vi "ReadHdrDates_LS1.vi"(7 "Data Folder Path":path, 8 "error in (no error)":errorcluster, 9 "Session":i32=-1, 10 "Date String":string="All" caption="Date String (yymmdd)", 11 "nombre (-1)":i32=-1) -> (0 "error out":errorcluster, 2 "Dates":string[](array[string]), 3 "ScanParams":T1[](array[typedef]))   [LabVIEW 2010]
doc: "Ce VI lit les données contenu dans le fichier de sauvegarde automatique. Ces données correspondent aux valeurs prises lors du dernier balayage. La sauvegarde automatique est effectué après chaque acquisition."
uses:
  Interface Class/ScanParams.ctl
  Interface Class/Interface.lvclass
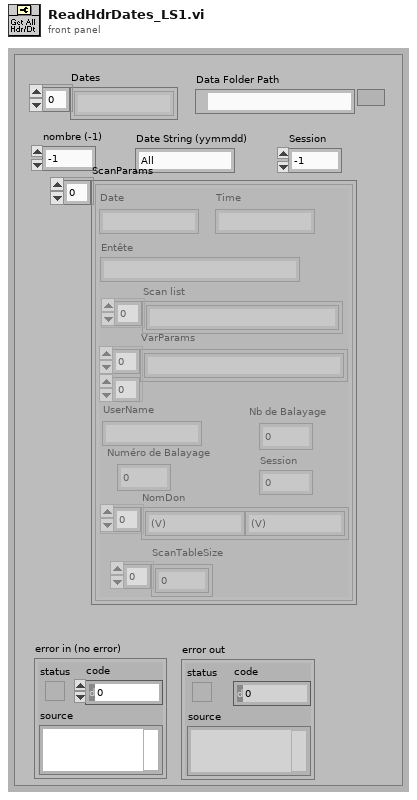
[diagram p1: front panel]
types:
  T1 = typedef "Interface.lvclass/ScanParams.ctl" = cluster{"Entête":string, "Scan list":string[], "NbCourbe":i32, "IndCourbe":i64, "NomDon":string[], "Session ":i32, "Date":string, "Time":string, "VarParams":string[][], "UserName":string, "ScanTableSize":i32[]}
  T2 = enum16{"open", "replace", "create", "open or create", "replace or create", "replace or create with confirmation"}
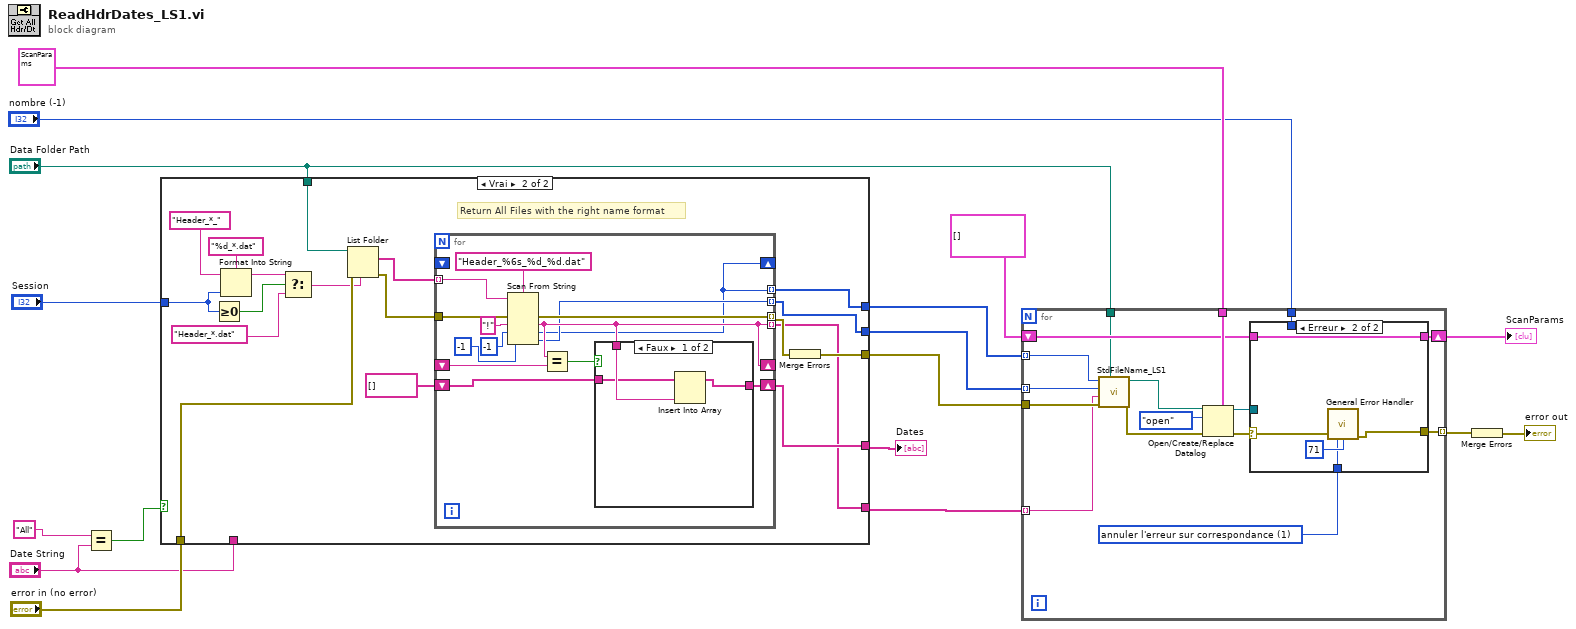
[diagram p0: block diagram]
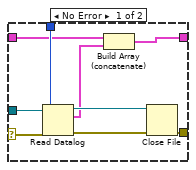
[diagram p2: hidden frame]
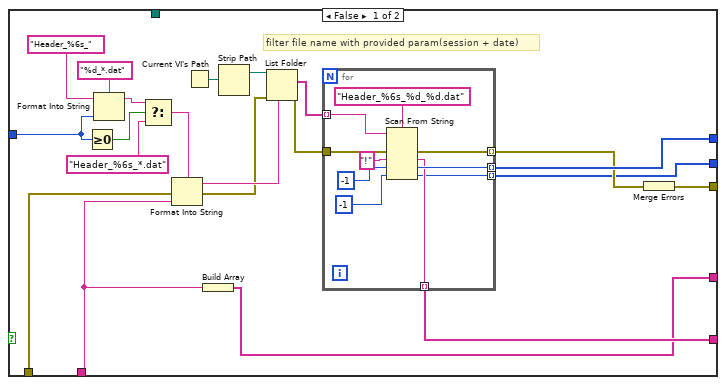
[diagram p3: hidden frame]
diagram:
  n1 = Equal?(x="All" ("Date String"), y="Date String") -> (x = y?=w8:bool)
  n2 = case shown="Vrai" w8 {
    tunnel: "error in (no error)" -> [w36 w66]
    tunnel: [w31 w61] -> w11
    tunnel: [w30 w64] -> w14
    tunnel: "Date String" -> [w27 _]
    tunnel: [w28 w59] -> w6
    tunnel: [w26 w60] -> w5
    tunnel: "Session" -> [w21 w54]
    tunnel: [w18 w50] -> w3
    tunnel: "Data Folder Path" -> [_ w49]
    frame False {
      # "filter file name with provided param(session + date)"
      n3 = Greater Or Equal To 0?(x=w21) -> (x >= 0?=w22:bool)
      n4 = Format Into String(format string="%d_*.dat" ("filtre"), initial string="Header_%6s_" ("filtre"), w21) -> (resulting string=w24:string)  [unwired: 1 in, 1 out]
      n5 = Select(t=w24, s=w22, f="Header_%6s_*.dat" ("filtre")) -> (s? t:f=w20:string)
      n6 = Format Into String(format string=w20, error in=w36, w27) -> (resulting string=w35:string, error out=w34:errorcluster)  [unwired: 1 in]
      n7 = Current VI's Path() -> (path=w38:path)
      n8 = Build Array(w27) -> (w26:string[])
      n9 = Strip Path(path=w38) -> (stripped path=w37:path)  [unwired: 1 out]
      n10 = List Folder(path=w37, pattern=w35, error in=w34) -> (filenames=w33:string[], error out=w32:errorcluster)  [unwired: 1 in, 2 out]
      n11 = for {
        tunnel: w33 -> [w48] mode=indexing
        tunnel: w32 -> [w47]
        tunnel: [w46] -> w29 mode=indexing
        tunnel: [w43] -> w31 mode=indexing
        tunnel: [w42] -> w28 mode=indexing
        tunnel: [w40] -> w18 mode=indexing
        n12 = Scan From String(format string="Header_%6s_%d_%d.dat" ("chaîne de format"), input string=w48, error in=w47, default 1="!" ("valeur par défaut 1"), default 2=-1 ("Session"), default 3=i64 -1 ("valeur par défaut 3")) -> (error out=w46:errorcluster, output 1=w42:string, output 2=w43:i32, output 3=w40:i64)  [unwired: 1 in, 2 out]
      }
      n13 = Merge Errors(w29) -> (w30:errorcluster)
    }
    frame True {
      # "Return All Files with the right name format"
      n14 = Greater Or Equal To 0?(x=w54) -> (x >= 0?=w55:bool)
      n15 = Format Into String(format string="%d_*.dat" ("filtre"), initial string="Header_*_" ("filtre"), w54) -> (resulting string=w56:string)  [unwired: 1 in, 1 out]
      n16 = Select(t=w56, s=w55, f="Header_*.dat" ("filtre")) -> (s? t:f=w52:string)
      n17 = List Folder(path=w49, pattern=w52, error in=w66) -> (filenames=w65:string[], error out=w51:errorcluster)  [unwired: 1 in, 2 out]
      n18 = for {
        tunnel: w65 -> [w80] mode=indexing
        tunnel: w51 -> [w79]
        tunnel: [w78] -> w63 mode=indexing
        shift-right: [w70] -> _
        shift-left: _ -> [w73]
        shift-right: [w71] -> w60
        shift-left: string[] [] ("tableau") -> [w72]
        tunnel: [w68] -> w61 mode=indexing
        tunnel: [w70] -> w59 mode=indexing
        tunnel: [w69] -> w50 mode=indexing
        shift-right: [w68] -> _
        shift-left: _ -> [_]
        n19 = Scan From String(format string="Header_%6s_%d_%d.dat" ("chaîne de format"), input string=w80, error in=w79, default 1="!" ("valeur par défaut 1"), default 2=-1 ("Session"), default 3=i64 -1 ("Session")) -> (error out=w78:errorcluster, output 1=w70:string, output 2=w68:i32, output 3=w69:i64)  [unwired: 1 in, 2 out]
        n20 = Equal?(x=w70, y=w73) -> (x = y?=w74:bool)
        n21 = case shown="Faux" w74 {
          tunnel: w70 -> [w83 _]
          tunnel: w72 -> [w82 w84]
          tunnel: [w81 w84] -> w71
          frame False {
            n22 = Insert Into Array(array=w82, new element=w83) -> (w81:string[])  [unwired: 1 in]
          }
          frame True {
          }
        }
      }
      n23 = Merge Errors(w63) -> (w64:errorcluster)
    }
  }
  "Dates" <- w5
  n24 = for {
    tunnel: [w100] -> w13 mode=indexing
    tunnel: T1 {"Entête"="", "Scan list"=[], "NbCourbe"=1, "IndCourbe"=1, "NomDon"=["RTêta;", "X&Y;"], "Session "=0, "Date"="", "Time"="", "VarParams"=[], "UserName"="", "ScanTableSize"=[]} ("ScanParams") -> [w99]
    tunnel: w6 -> [w89] mode=indexing
    tunnel: "nombre (-1)" -> [w94]
    tunnel: w14 -> [w93]
    tunnel: w11 -> [w92] mode=indexing
    shift-right: [w90] -> w2
    shift-left: T1[] [] -> [w91]
    tunnel: w3 -> [w88] mode=indexing
    tunnel: "Data Folder Path" -> [w87]
    w85 = 1 items=["pas d'exception", "annuler l'erreur sur correspondance", "définir l'erreur sur correspondance"] ("[exception action] (none:0)")
    n25 = call "StdFileName_LS1.vi"("chemin de base"=w87, "error in (no error)"=w93, "Date"=w89, "Scan"=w88, "Session"=w92) -> ("error out"=w97:errorcluster, "chemin Headers"=w98:path)  [unwired: 2 in, 3 out]
    n26 = Open/Create/Replace Datalog(5:w99, 8:w97, 10:T2."open" ("opération (0 : open)"), 11:w98) -> (0:w86:errorcluster, 3:w96:refnum<k1>)  [unwired: 2 in, 1 out]
    n27 = case shown="Erreur" w86 {
      selector: w86 -> [w101 w113]
      tunnel: [w109 w112] -> w100
      tunnel: w96 -> [w108 _]
      tunnel: w94 -> [w105 _]
      tunnel: w91 -> [w104 w114]
      tunnel: [w103 w114] -> w90
      tunnel: w85 -> [_ w110]
      frame No Error {
        n28 = Read Datalog(4:w101, 6:w105, 7:w108) -> (0:w107:errorcluster, 2:w102:T1[], 3:w106:refnum<k1>)
        n29 = Build Array (concatenate)(w104, w102) -> (w103:T1[])
        n30 = Close File(refnum=w106, error in=w107) -> (error out=w109:errorcluster)  [unwired: 1 out]
      }
      frame Error {
        n31 = call <vilib>:"General Error Handler.vi"("error in (no error)"=w113, "[exception action] (none:0)"=w110, "[exception code]"=71) -> ("error out"=w112:errorcluster)  [unwired: 8 in, 4 out]
      }
    }
  }
  "ScanParams" <- w2
  n32 = Merge Errors(w13) -> (→"error out":errorcluster)
